vi "Real SVD Factorization.vi"(0 "A":T1) -> (1 "U":T1, 2 "S":dbl[](array[numeric]) format="%.2f", 3 "V":T1, 4 "error":i32)   [LabVIEW 2017, in "NI_AALPro.lvlib"]
doc: "Performs the singular value decomposition (SVD) of a given m-by-n real matrix <B>A</B>. The dimentions of U, S, and V are m x min(m, n), min(m, n), and n x min(m, n), respectively."
uses:
  <vilib>/Analysis/NI_AALPro.lvlib
  <vilib>/Analysis/Matrix/Datatypes/RealMatrix.ctl
  <resource>/lvanlys.dll
  <vilib>/Analysis/Matrix/NI_Matrix.lvlib
panel:
  # "SVD Factorization"
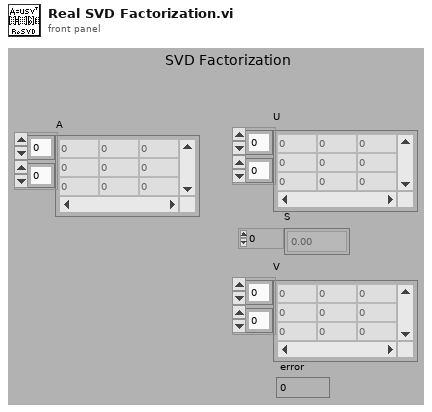
[diagram p1: front panel]
types:
  T1 = typedef "NI_Matrix.lvlib/RealMatrix.ctl" = dbl[][]
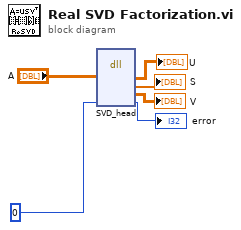
[diagram p0: block diagram]
diagram:
  n1 = dll-call lib="e:/builds/penguin/labview/branches/2017/dev/dist/resource/lvanlys.*" fn="SVD_head"("A"="A", 0) -> ("A"=→"U":T1, "S"=→"S":dbl[], "V"=→"V":T1, →"error":i32)  [unwired: 6 in, 2 out]
